vi "Expand.vi"(8 "error in (no error)":errorcluster, 10 "ToExpand in":refnum<data-value>, 11 "PathTree in":refnum<class "RouteTree.lvclass">) -> (0 "error out":errorcluster, 1 "ExpandedSearchNodes":refnum<data-value>[](array[refnum]), 2 "ToExpand out":refnum<data-value>, 3 "PathTree out":refnum<class "RouteTree.lvclass">)   [LabVIEW 2009, in "RouteTree.lvclass"]
uses:
  RouteTree.lvclass
  TreeNode/TreeNode.lvclass
  Waypoint/Waypoint.lvclass
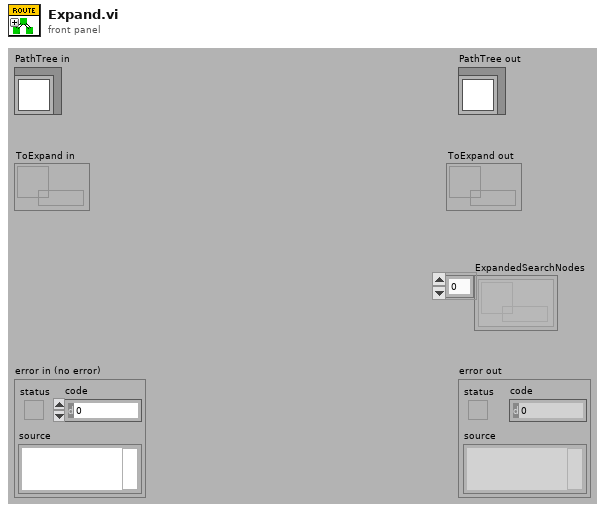
[diagram p1: front panel]
types:
  T1 = typedef "Waypoint.lvclass/point.ctl" = cluster{"X":dbl, "Y":dbl}
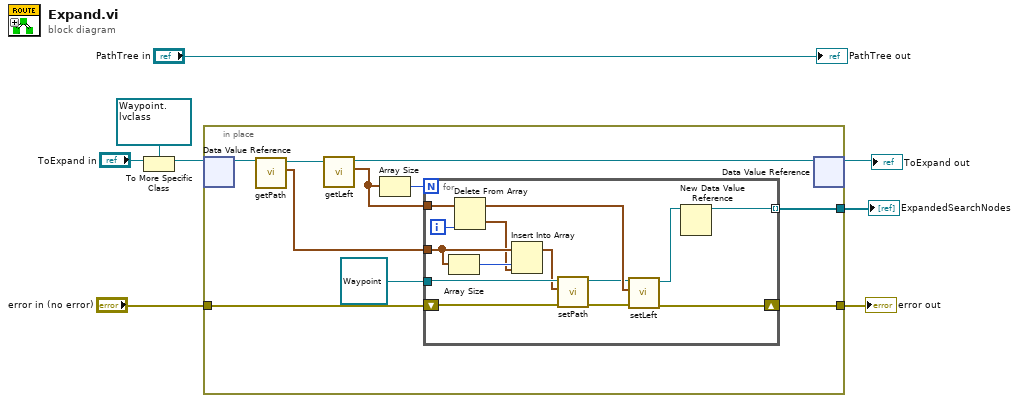
[diagram p0: block diagram]
diagram:
  n1 = To More Specific Class(target class=refnum<data-value> refnum ("data value reference"), reference="ToExpand in") -> (specific class reference=w2:refnum<data-value>)  [unwired: 1 in, 1 out]
  n2 = in-place {
    in-place-border: [w17] -> w7
    in-place-border: [w16] -> w6
    in-place-border: "error in (no error)" -> [w15]
    n3 = in-place-dvr #1(w2) -> (w12:refnum<class "Waypoint.lvclass">)  [unwired: 1 out]
    n4 = call "getPath.vi"("Waypoint in"=w12) -> ("Path"=w9:T1[], "Waypoint out"=w11:refnum<class "Waypoint.lvclass">)  [unwired: 8 in, 1 out]
    n5 = call "getLeft.vi"("Waypoint in"=w11) -> ("left"=w13:T1[], "Waypoint out"=w10:refnum<class "Waypoint.lvclass">)  [unwired: 8 in, 1 out]
    n6 = Array Size(array=w13) -> (size(s)=w18:i32)
    n7 = for {
      N: w18 -> [_]
      tunnel: w13 -> [w32]
      tunnel: [w20] -> w17 mode=indexing
      shift-right: [w19] -> w16
      shift-left: w15 -> [w23]
      tunnel: refnum<class "Waypoint.lvclass"> refnum ("Waypoint.lvclass") -> [w25]
      tunnel: w9 -> [w29]
      i -> [w31]
      n8 = Array Size(array=w29) -> (size(s)=w28:i32)
      n9 = Delete From Array(array=w32, index=w31) -> (deleted portion=w27:T1, array with subset deleted=w30:T1[])  [unwired: 1 in]
      n10 = Insert Into Array(array=w29, index=w28, new element=w27) -> (w24:T1[])
      n11 = call "setPath.vi"("error in (no error)"=w23, "Path"=w24, "Waypoint in"=w25) -> ("error out"=w22:errorcluster, "Waypoint out"=w26:refnum<class "Waypoint.lvclass">)  [unwired: 7 in]
      n12 = call "setLeft.vi"("error in (no error)"=w22, "left"=w30, "Waypoint in"=w26) -> ("error out"=w19:errorcluster, "Waypoint out"=w21:refnum<class "Waypoint.lvclass">)  [unwired: 7 in]
      n13 = New Data Value Reference(data value=w21) -> (data value reference=w20:refnum<data-value>)  [unwired: 1 in, 1 out]
    }
    n14 = in-place-dvr #1(w10) -> (→"ToExpand out":refnum<data-value>)  [unwired: 1 out]
  }
  "error out" <- w6
  "ExpandedSearchNodes" <- w7
  "PathTree out" <- "PathTree in"
